vi "XVC_SERVER_UDPV2.vi"() -> ()   [LabVIEW 2017]
panel:
  out "connection ID 2":refnum<k16>
  out "port":refnum<k16>
  out "字符串 4":string
  out "字符串 3":string
  out "字符串 2":string
  out "error out":errorcluster={"status"=TRUE, "code"=56, "source"="TCP Listen.vi:7210001->XVC_SERVER_UDPV2.vi中的等待TCP侦听器"} caption="错误输出"
  out "连接的字符串":string
  out "错误输出 5":errorcluster caption="错误输出"
  out "错误输出 4":errorcluster caption="错误输出"
  in  "字符串":string=":\u0005\u0000\u0000\u0000\u001f\u0000"
  out "错误输出 3":errorcluster={"status"=TRUE, "code"=56, "source"="TCP Listen.vi:7210001->XVC_SERVER_UDPV2.vi中的等待TCP侦听器"} caption="错误输出"
  out "错误输出 2":errorcluster={"status"=TRUE, "code"=66, "source"="XVC_SERVER_UDP.vi中的读取TCP数据"} caption="错误输出"
  out "错误输出":errorcluster
  out "x+1":u32=3558
  in  "data out 5":string="shift:\u0005\u0000\u0000\u0000ÿ\u0000"
  in  "address":string="192.168.10.20"
  out "data out 3":string
  in  "data out 2":string="shift"
  out "x != 0?":bool
  in  "Client Closed":string="The client VI closed the connection."
  in  "Stop":bool
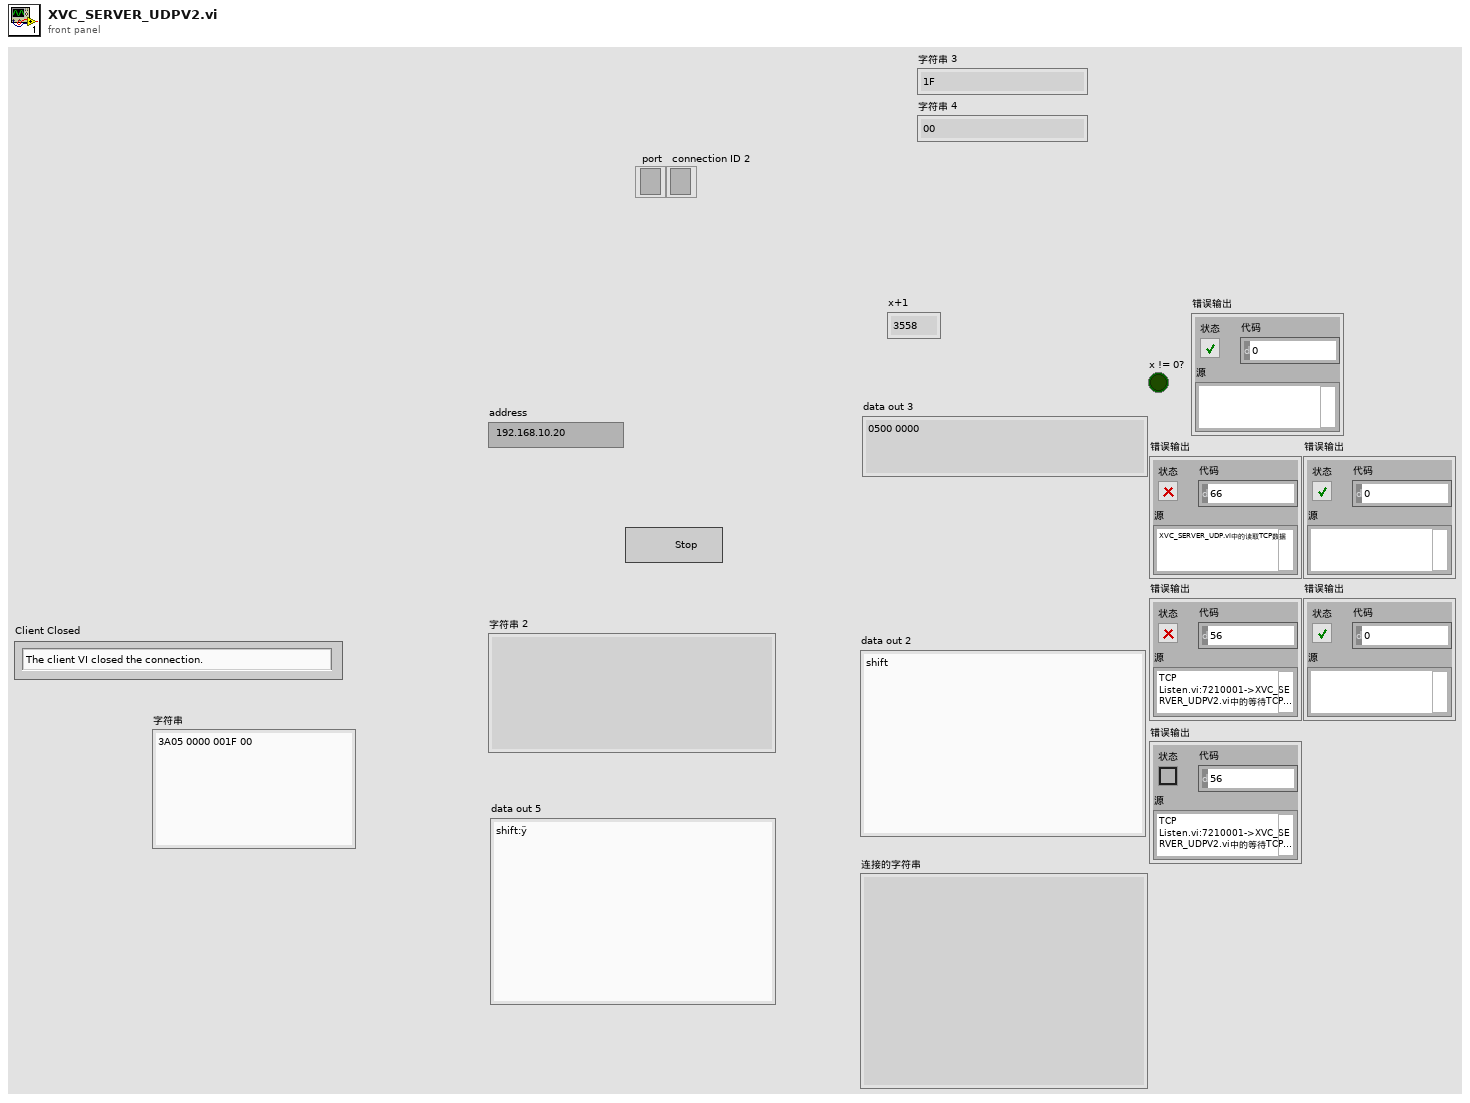
[diagram p1: front panel]
types:
  T1 = enum16{"Standard", "Buffered", "CRLF", "Immediate"}
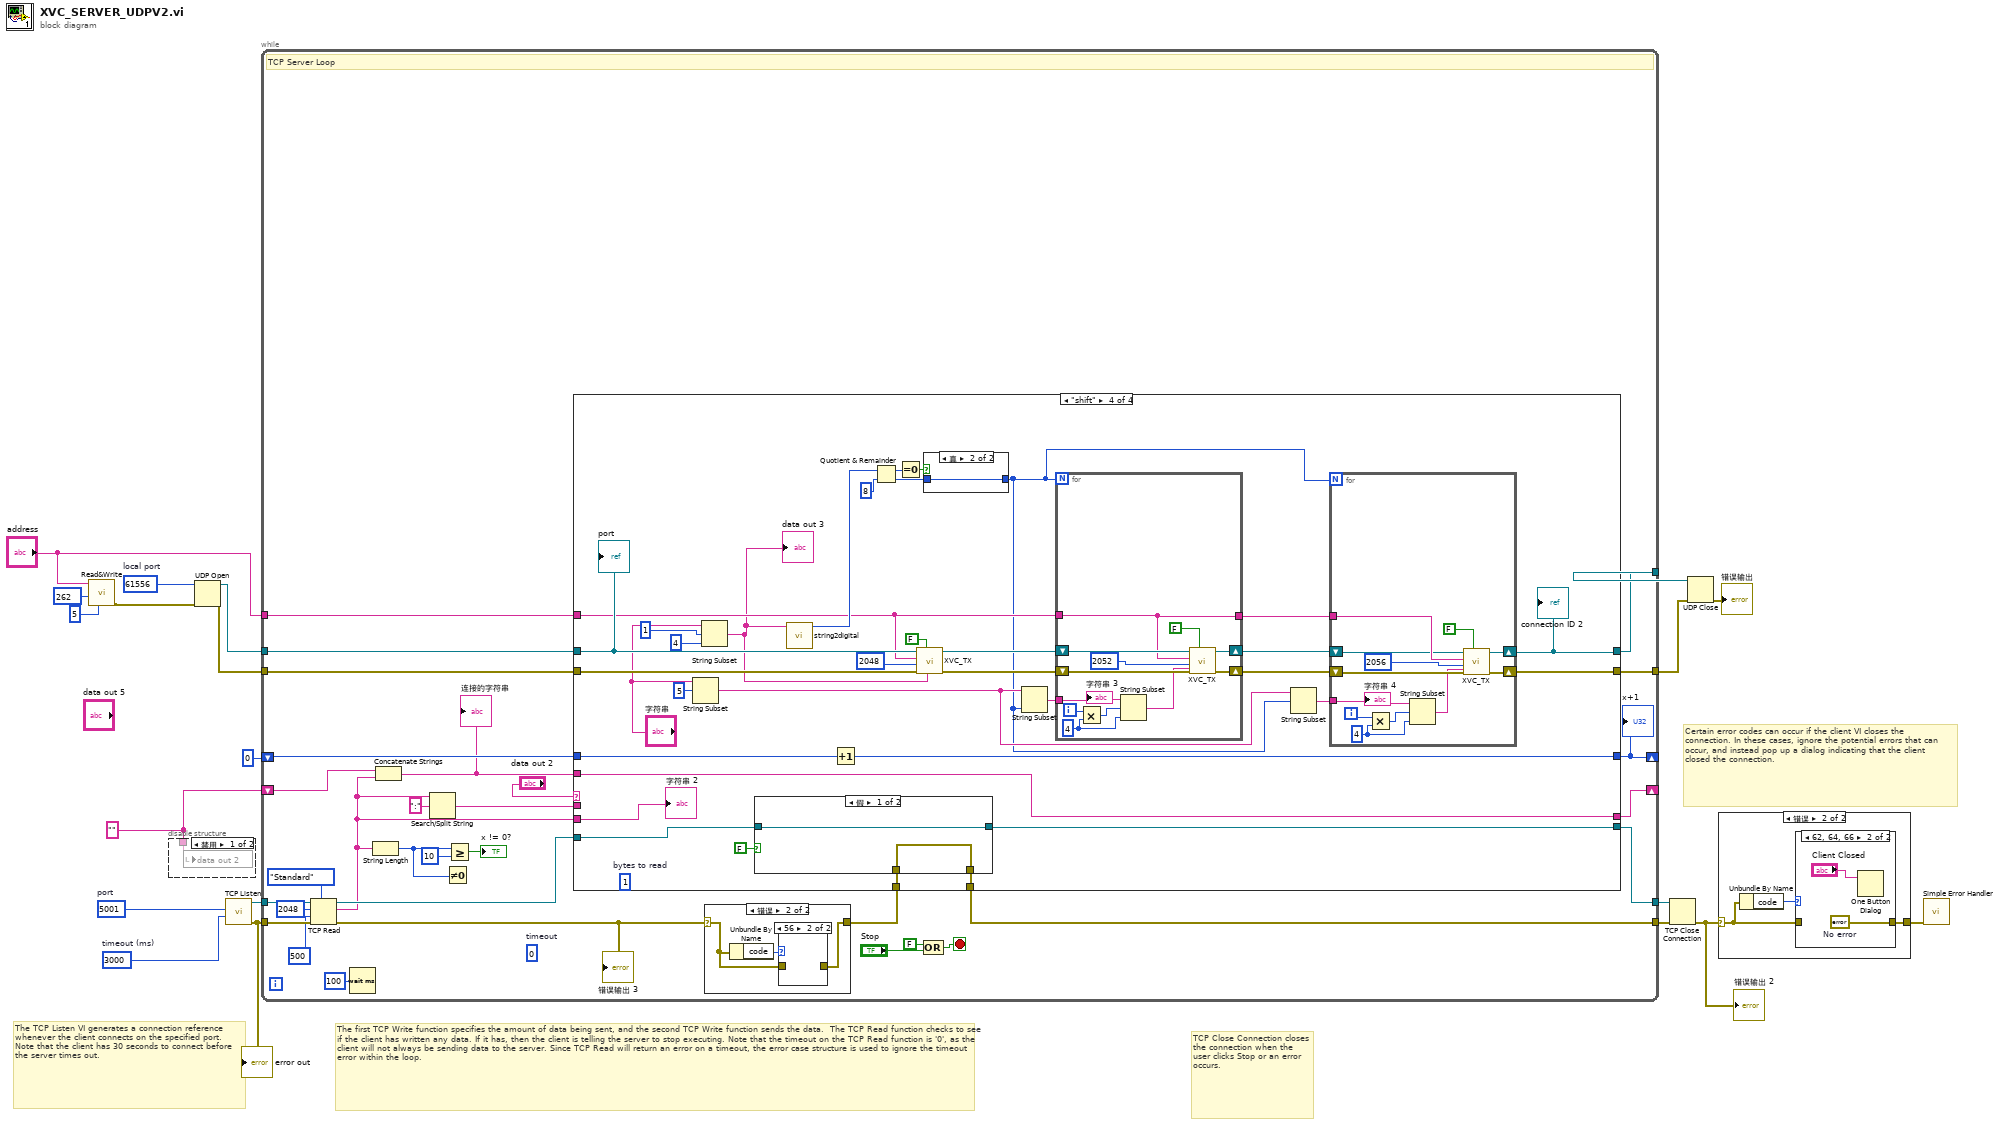
[diagram p0: block diagram]
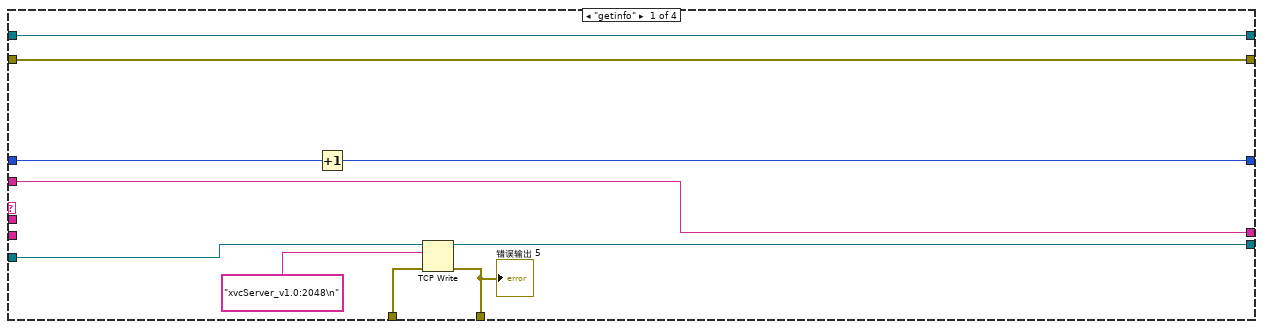
[diagram p5: hidden frame]
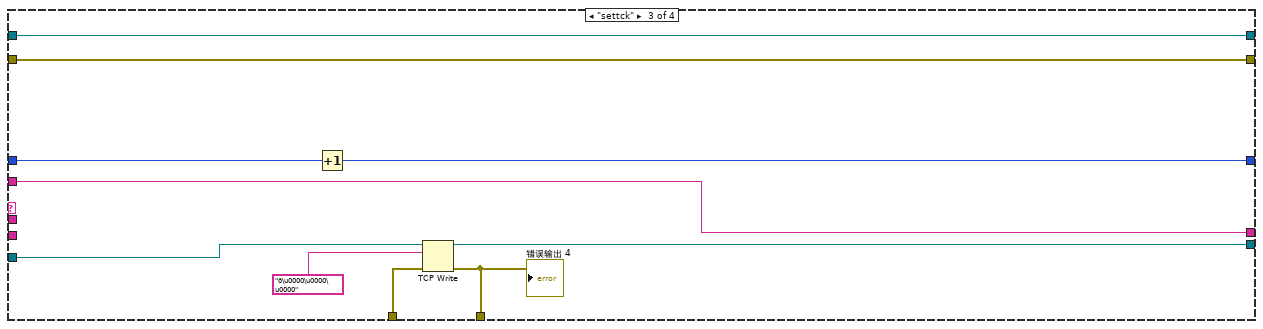
[diagram p7: hidden frame]
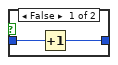
[diagram p8: hidden frame]
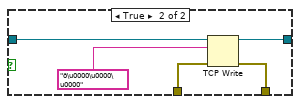
[diagram p9: hidden frame]
diagram:
  w12 = u16 61556  # local port
  w8 = ""
  w13 = u16 5001  # port
  w14 = 3000  # timeout (ms)
  # "TCP Close Connection closes the connection when the user clicks Stop or an error occurs."
  # "The TCP Listen VI generates a connection reference whenever the client connects on the specified port. Note that the client has 30 seconds to connect before the server times out."
  # "Certain error codes can occur if the client VI closes the connection. In these cases, ignore the potential errors that can occur, and instead pop up a dialog indicating that the client closed the connection."
  # "The first TCP Write function specifies the amount of data being sent, and the second TCP Write function sends the data.  The TCP Read function checks to see if the client has written any data. If it has, then the client is telling the server to stop executing. Note that the timeout on the TCP Read function is '0', as the client will not always be sending data to the server. Since TCP Read will return an error on a timeout, the error case structure is used to ignore the timeout error within the loop."
  n1 = call "Read&Write.vi"("In"=u8 5, "Address"=u32 262, "address"="address") -> ("error out"=w9:errorcluster)  [unwired: 7 in, 1 out]
  n2 = disable-structure shown="禁用" {
    disable-tunnel: w8 -> [w21 _]
    frame Disabled {
      n3 = local write "data out 2"(w21) -> ()
    }
    frame Enabled {
    }
  }
  n4 = UDP Open(8:w9, 11:w12) -> (port=w4:refnum<k16>, 0:w3:errorcluster)  [unwired: 3 in, 1 out]
  n5 = call <vilib>:"TCP Listen.vi"("timeout ms (wait forever: -1)"=w14, "port"=w13) -> ("error out"=w15:errorcluster, "connection ID"=w16:refnum<k5>)  [unwired: 5 in, 3 out]
  "error out" <- w15
  n6 = while {
    tunnel: [w38] -> w19
    tunnel: [w36] -> w20
    tunnel: w16 -> [w52]
    tunnel: w15 -> [w49]
    shift-right: [w35] -> _
    shift-left: w8 -> [w44]
    shift-right: [w32] -> _
    shift-left: u32 0 -> [w34]
    tunnel: "address" -> [w31]
    tunnel: w4 -> [w30]
    tunnel: w3 -> [w29]
    tunnel: [w28] -> w2
    tunnel: [w27] -> w1
    stop <- w50 stop-if-true
    (unwired) 0  # timeout
    (unwired) 1  # bytes to read
    # "TCP Server Loop"
    n7 = TCP Read(connection ID=w52, bytes to read=2048, error in (no error)=w49, 7:T1."Standard" ("mode (standard)"), 9:500 ("timeout ms (25000)")) -> (connection ID out=w37:refnum<k5>, data out=w22:string, error out=w47:errorcluster)
    "错误输出 3" <- w47
    n8 = Wait (ms)(milliseconds to wait=u32 100) -> ()  [unwired: 1 out]
    n9 = String Length(string=w22) -> (length=w42:i32)
    n10 = Concatenate Strings(w44, w22) -> (w26:string)
    "连接的字符串" <- w26
    n11 = Search/Split String(string=w22, search string/char (-)=":" ("正则表达式")) -> (match + rest of string=w24:string)  [unwired: 1 in, 2 out]
    n12 = Not Equal To 0?(x=w42) -> ()  [unwired: 1 out]
    n13 = Greater Or Equal?(x=w42, y=10) -> (x >= y?=→"x != 0?":bool)
    n14 = case shown="错误" w47 {
      selector: w47 -> [w148 w150]
      tunnel: [w148 w149] -> w39
      frame No Error {
      }
      frame Error {
        n15 = Unbundle By Name(w150) -> ("code"=w151:i32)
        n16 = case shown="56" w151 {
          tunnel: w150 -> [w152 _]
          tunnel: [w152 _] -> w149
          frame Default {
          }
          frame 56 {
          }
        }
      }
    }
    n17 = case shown="\"shift\"" "data out 2" {
      tunnel: w37 -> [w62 w65 w78 w113]
      tunnel: w39 -> [w60 w64 w76 w112]
      tunnel: [w59 w64 w75 w111] -> w38
      tunnel: [w58 w65 w74 w110] -> w36
      tunnel: [w53 w63 w69 w101] -> w35
      tunnel: [w57 w66 w73 w109] -> w32
      tunnel: w34 -> [w56 w66 w72 w108]
      tunnel: w31 -> [_ _ _ w93]
      tunnel: w30 -> [w55 w68 w71 w97]
      tunnel: w29 -> [w54 w67 w70 w95]
      tunnel: [w54 w67 w70 w83] -> w28
      tunnel: [w55 w68 w71 w84] -> w27
      tunnel: w26 -> [w53 w63 w69 w101]
      tunnel: w24 -> [_ _ _ _]
      tunnel: w22 -> [_ _ _ w100]
      frame "getinfo" {
        n18 = Increment(x=w56) -> (x+1=w57:u32)
        n19 = TCP Write(connection ID=w62, data in="xvcServer_v1.0:2048\n", error in (no error)=w60) -> (connection ID out=w58:refnum<k5>, error out=w59:errorcluster)  [unwired: 1 in, 1 out]
        "错误输出 5" <- w59
      }
      frame "x", Default {
      }
      frame "settck" {
        n20 = Increment(x=w72) -> (x+1=w73:u32)
        n21 = TCP Write(connection ID=w78, data in="ð\u0000\u0000\u0000", error in (no error)=w76) -> (connection ID out=w74:refnum<k5>, error out=w75:errorcluster)  [unwired: 1 in, 1 out]
        "错误输出 4" <- w75
      }
      frame "shift" {
        n22 = String Subset(string="字符串", offset (0)=5 ("偏移量(0)")) -> (substring=w80:string)  [unwired: 1 in]
        n23 = String Subset(string="字符串", offset (0)=1 ("length (rest)"), length (rest)=4 ("length (rest)")) -> (substring=w88:string)
        "data out 3" <- w88
        n24 = case shown="假" FALSE {
          tunnel: w113 -> [w142 w147]
          tunnel: w112 -> [w141 w145]
          tunnel: [w141 w144] -> w111
          tunnel: [w142 w143] -> w110
          frame False {
          }
          frame True {
            n25 = TCP Write(connection ID=w147, data in="ð\u0000\u0000\u0000", error in (no error)=w145) -> (connection ID out=w143:refnum<k5>, error out=w144:errorcluster)  [unwired: 1 in, 1 out]
          }
        }
        n26 = call "string2digital.vi"("data in"=w88) -> ("number"=w106:u32)  [unwired: 10 in]
        n27 = Increment(x=w108) -> (x+1=w109:u32)
        n28 = Quotient & Remainder(x=w106, y=u8 8) -> (x-y*floor(x/y)=w98:u32, floor(x/y)=w102:u32)
        n29 = Equal To 0?(x=w98) -> (x = 0?=w99:bool)
        n30 = call "XVC_TX.vi"("data in"=w88, "Read (TRUE)"=FALSE, "error in"=w95, "Address"=u32 2048, "IP address"=w93, "connection ID"=w97) -> ("error out"=w94:errorcluster, "connection ID 2"=w96:refnum<k16>)  [unwired: 3 in, 1 out]
        n31 = case shown="真" w99 {
          tunnel: [w127 w128] -> w79
          tunnel: w102 -> [w126 w128]
          frame False {
            n32 = Increment(x=w126) -> (x+1=w127:u32)
          }
          frame True {
          }
        }
        n33 = String Subset(string=w80, length (rest)=w79) -> (substring=w87:string)  [unwired: 1 in]
        n34 = for {
          N: w79 -> [_]
          tunnel: w93 -> [w135]
          shift-right: [w139] -> w85
          shift-left: w94 -> [w140]
          shift-right: [w137] -> w86
          shift-left: w96 -> [w138]
          tunnel: w87 -> [w130]
          tunnel: [w135] -> w82
          i -> [w132]
          w131 = 4 ("长度（剩余）")
          n35 = Multiply(x=w132, y=w131) -> (x*y=w133:i32)
          n36 = String Subset(string=w130, offset (0)=w133, length (rest)=w131) -> (substring=w129:string)
          n37 = call "XVC_TX.vi"("data in"=w129, "Read (TRUE)"=FALSE, "error in"=w140, "Address"=u32 2052, "IP address"=w135, "connection ID"=w138) -> ("error out"=w139:errorcluster, "connection ID 2"=w137:refnum<k16>)  [unwired: 3 in, 1 out]
          "字符串 3" <- w130
        }
        n38 = String Subset(string=w80, offset (0)=w79) -> (substring=w81:string)  [unwired: 1 in]
        n39 = for {
          N: w79 -> [_]
          tunnel: w82 -> [w125]
          shift-right: [w123] -> w83
          shift-left: w85 -> [w124]
          shift-right: [w121] -> w84
          shift-left: w86 -> [w122]
          tunnel: w81 -> [w114]
          i -> [w116]
          w117 = 4 ("长度（剩余）")
          n40 = Multiply(x=w116, y=w117) -> (x*y=w118:i32)
          n41 = String Subset(string=w114, offset (0)=w118, length (rest)=w117) -> (substring=w115:string)
          n42 = call "XVC_TX.vi"("data in"=w115, "Read (TRUE)"=FALSE, "error in"=w124, "Address"=u32 2056, "IP address"=w125, "connection ID"=w122) -> ("error out"=w123:errorcluster, "connection ID 2"=w121:refnum<k16>)  [unwired: 3 in, 1 out]
          "字符串 4" <- w114
        }
        "connection ID 2" <- w84
        "字符串 2" <- w100
        "port" <- w97
      }
    }
    "x+1" <- w32
    n43 = Compound Arithmetic op=OR(FALSE ("值"), "Stop") -> (w50:bool)
  }
  n44 = TCP Close Connection(connection ID=w20, error in (no error)=w19) -> (error out=w18:errorcluster)  [unwired: 2 out]
  "错误输出 2" <- w18
  n45 = UDP Close(connection ID=w1, 8:w2) -> (error out=→"错误输出":errorcluster)  [unwired: 1 out]
  n46 = case shown="错误" w18 {
    selector: w18 -> [w153 w155]
    tunnel: [w153 w154] -> w17
    frame No Error {
    }
    frame Error {
      n47 = Unbundle By Name(w155) -> ("code"=w156:i32)
      n48 = case shown="62, 64, 66" w156 {
        tunnel: w155 -> [w157 _]
        tunnel: [w157 w159] -> w154
        frame Default {
        }
        frame 62, 64, 66 {
          w159 = errorcluster {"status"=FALSE, "code"=0, "source"=""}  # No error
          n49 = One Button Dialog(message="Client Closed") -> ()  [unwired: 1 in, 1 out]
        }
      }
    }
  }
  n50 = call <vilib>:"Simple Error Handler.vi"("error in (no error)"=w17) -> ()  [unwired: 1 in, 8 out]
